vi "Read AI.vi"(8 "error in":errorcluster, 11 "DAQmx in":refnum<class "DAQmx.lvclass">) -> (0 "error out":errorcluster, 2 "AI []":waveform(dbl)[](array[waveform]), 3 "DAQmx out":refnum<class "DAQmx.lvclass">, 4 "AI time (ms)":u32=2)   [LabVIEW 2019, in "DAQmx.lvclass"]
uses:
  DAQmx.lvclass
  <resource>/objmgr/daqmx.rc
  Instrument.DAQ/Instrument.DAQ.lvclass
  Instrument.DAQ/Waveguide Model/Waveguide Model--Cluster.ctl
  <vilib>/Waveform/WDTOps.llb/WDT Append Waveforms DBL.vi
  <vilib>/DAQmx/read.llb/DAQmx Read (Analog 1D Wfm NChan NSamp).vi
panel:
  out "Available Samples":u32[][](graph)
  in  "show graph?":bool
  out "Ratio Chart":u32[][](graph)
  out "Waveform Graph":waveform(dbl)[](graph)
  out "P Check":bool[](array[boolean])
  out "Numeric":i32
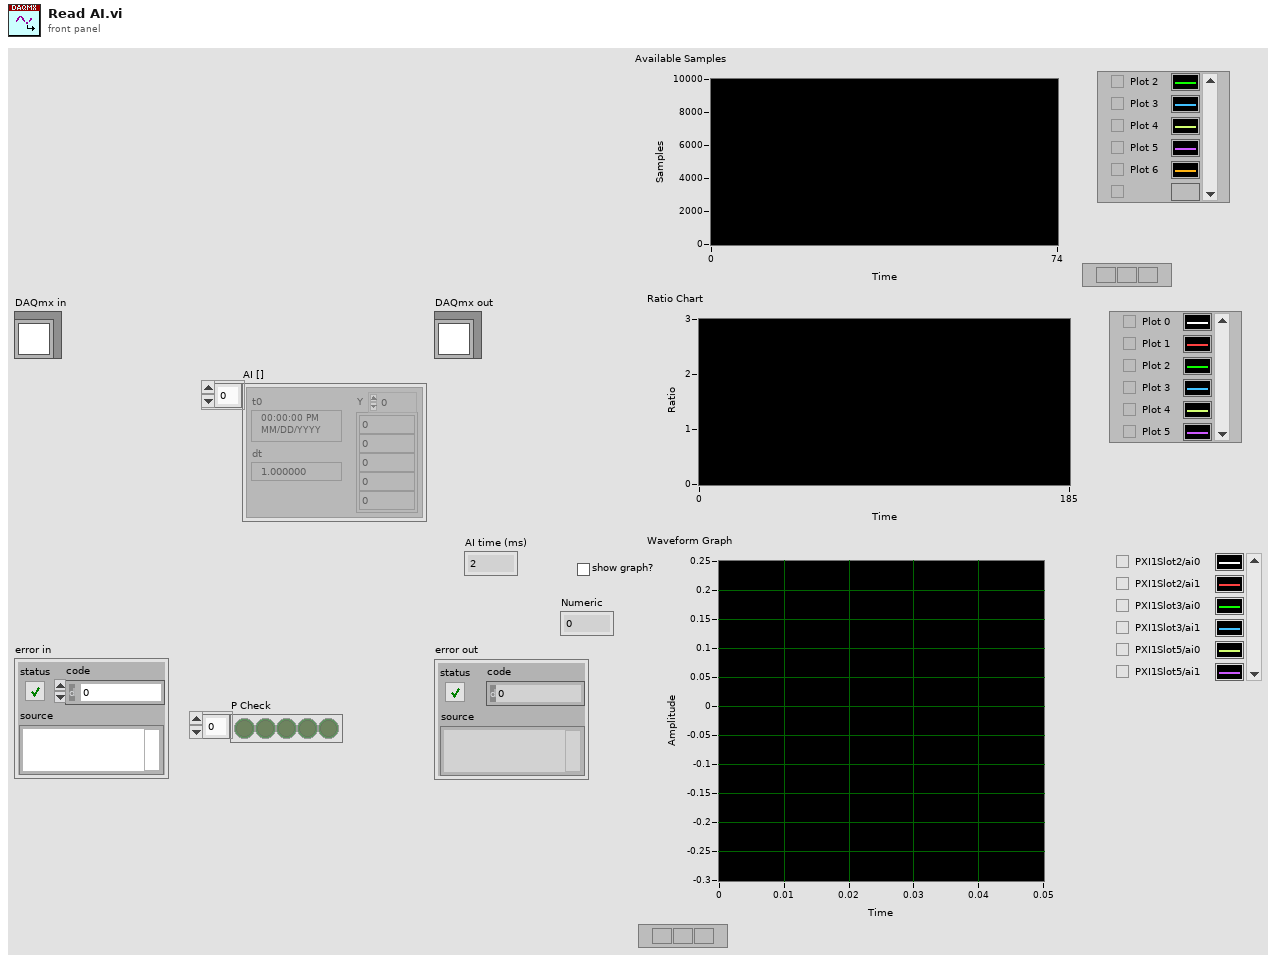
[diagram p1: front panel]
types:
  T1 = typedef "Instrument.Lockin.lvlib/Instrument.DAQ.lvclass/Waveguide Model--Cluster.ctl" = cluster{"Vsource Index":i32, "Vsg Index":i32, "V+":i32, "V-":i32}
  T2 = typedef "DAQmx.lvclass/DAQ.Config.AI--Cluster--Array.ctl" = T3[]
  T3 = typedef "DAQmx.lvclass/DAQ.Config.AI--Cluster.ctl" = cluster{"Channels":tag, "Coupling":T4, "Range":T5, "input terminal configuration":i32, "Type":T6}
  T4 = typedef "DAQmx.lvclass/DAQ.Config.AI.Coupling--enum.ctl" = u16
  T5 = typedef "DAQmx.lvclass/DAQ.Config.AI.Range--enum.ctl" = enum16{"±0.316", "±1.00", "±3.16", "±10.0", "±31.6", "±42.4", ""}
  T6 = typedef "DAQmx.lvclass/DAQ.Config.Device Type--enum.ctl" = enum16{"None", "USB-4431", "PXI-446x"}
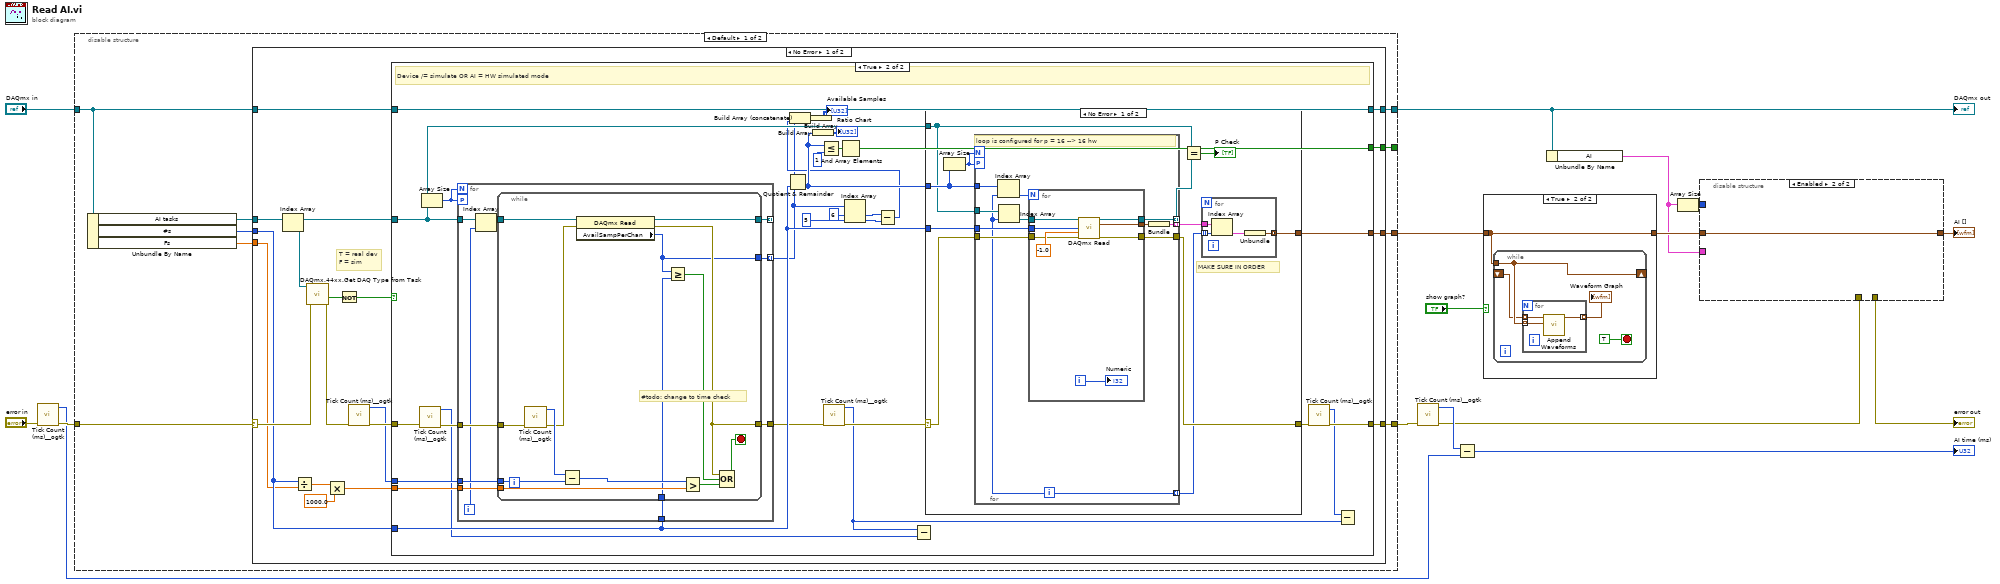
[diagram p0: block diagram]
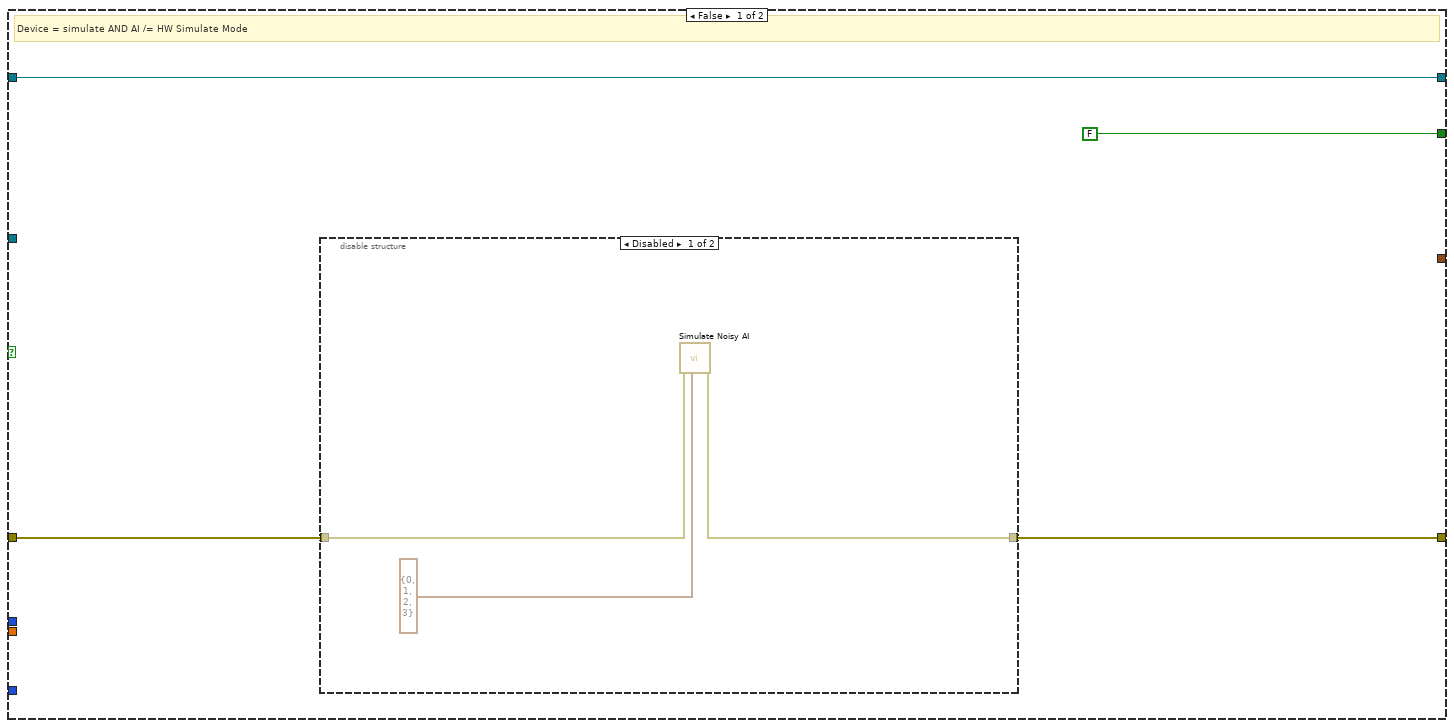
[diagram p2: hidden frame]
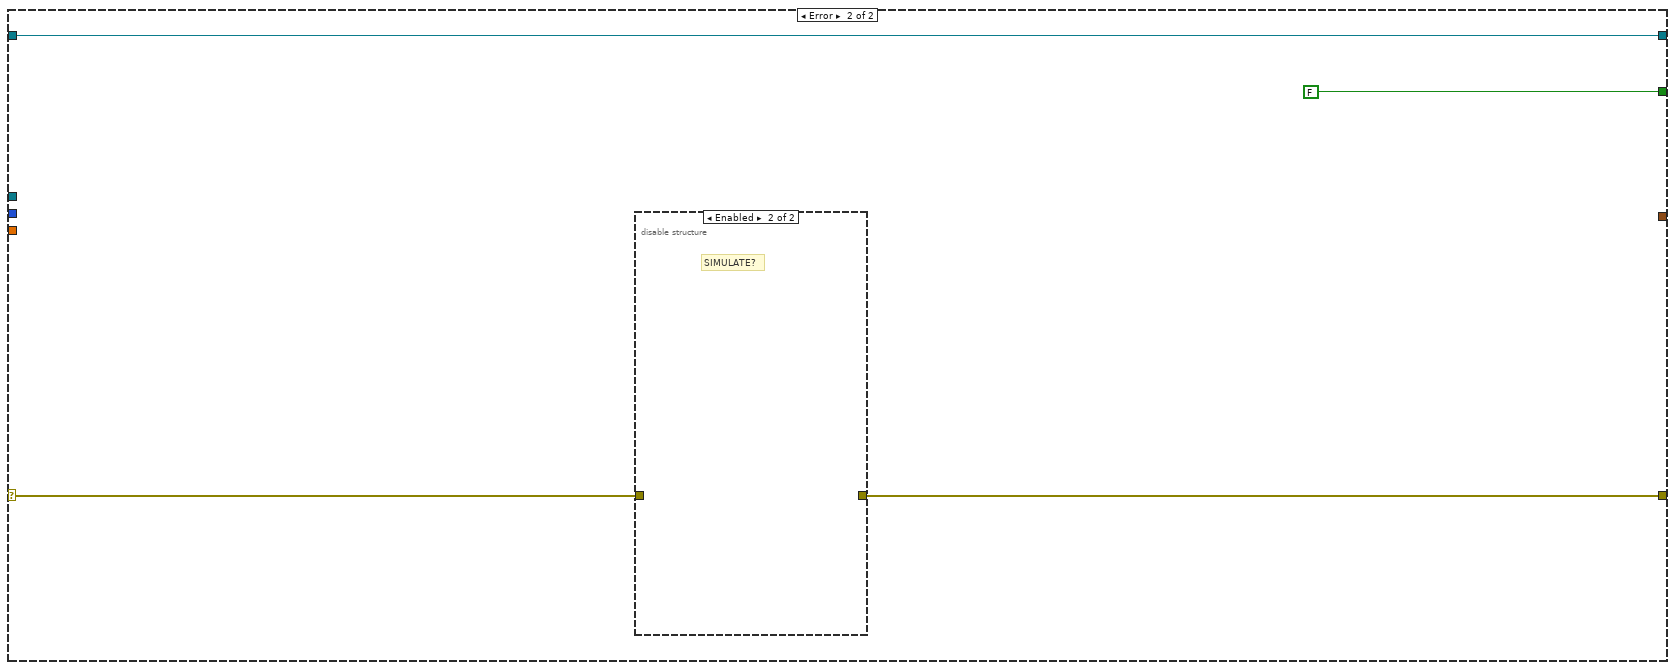
[diagram p5: hidden frame]
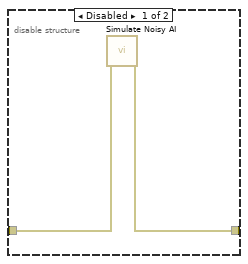
[diagram p6: hidden frame]
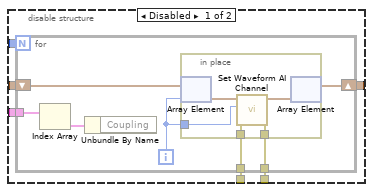
[diagram p8: hidden frame]
diagram:
  n1 = call <userlib>:"Tick Count (ms)__ogtk.vi"("error in (no error)"="error in") -> ("error out"=w15:errorcluster, "millisecond timer value"=w11:u32)  [unwired: 9 in]
  n2 = disable-structure shown="Default" {
    disable-tunnel: [w24 w146] -> w10
    disable-tunnel: "DAQmx in" -> [w23 w145]
    disable-tunnel: w15 -> [w20 w146]
    disable-tunnel: [w22 w145] -> w2
    disable-tunnel: [w19 _] -> _
    disable-tunnel: [w18 _] -> w3
    frame condition #0 (active) {
      n3 = Unbundle By Name(w23) -> ("AI tasks"=w21:refnum<k21>[], "#s"=w25:i32, "Fs"=w17:dbl)
      n4 = case shown="No Error" w20 {
        selector: w20 -> [w41 w141]
        tunnel: w25 -> [w40 _]
        tunnel: [w42 w142] -> w24
        tunnel: w21 -> [w32 _]
        tunnel: w23 -> [w43 w139]
        tunnel: [w30 w139] -> w22
        tunnel: w17 -> [w39 _]
        tunnel: [w29 FALSE] -> w19
        tunnel: [w28 _] -> w18
        frame No Error {
          # "T = real dev\nF = sim"
          n5 = Index Array(array=w32) -> (element=w26:refnum<k21>)  [unwired: 1 in]
          n6 = Divide(x=w40, y=w39) -> (x/y=w38:dbl)
          n7 = call "DAQmx.44xx.Get DAQ Type from Task.vi"("error in (no error)"=w41, "Task in"=w26) -> ("error out"=w35:errorcluster, "DevIsSimulated"=w31:bool)  [unwired: 6 in, 2 out]
          n8 = Multiply(x=w38, y=1000.0) -> (x*y=w34:dbl)
          n9 = Not(x=w31) -> (.not. x?=w27:bool)
          n10 = call <userlib>:"Tick Count (ms)__ogtk.vi"("error in (no error)"=w35) -> ("error out"=w36:errorcluster, "millisecond timer value"=w33:u32)  [unwired: 9 in]
          n11 = case shown="True" w27 {
            tunnel: w40 -> [_ w79]
            tunnel: w36 -> [w47 w77]
            tunnel: [w46 w78] -> w42
            tunnel: w43 -> [w44 w52]
            tunnel: w34 -> [_ w76]
            tunnel: w33 -> [_ w75]
            tunnel: w32 -> [_ w74]
            tunnel: [w44 w52] -> w30
            tunnel: [FALSE w73] -> w29
            tunnel: [_ w51] -> w28
            frame False {
              # "Device = simulate AND AI /= HW Simulate Mode"
              n12 = disable-structure shown="Disabled" {
                disable-tunnel: w47 -> [w49 _]
                disable-tunnel: [w48 _] -> w46
                frame Disabled {
                  n13 = call "Simulate Noisy AI.vi"("Waveguide Cluster"=T1 {"Vsource Index"=0, "Vsg Index"=1, "V+"=2, "V-"=3}, "error in (no error)"=w49) -> ("error out"=w48:errorcluster)  [unwired: 7 in, 2 out]
                }
                frame Enabled {
                  # "SIMULATE"
                }
              }
            }
            frame True {
              # "Device /= simulate OR AI = HW simulated mode"
              n14 = call <userlib>:"Tick Count (ms)__ogtk.vi"("error in (no error)"=w77) -> ("error out"=w72:errorcluster, "millisecond timer value"=w68:u32)  [unwired: 9 in]
              n15 = Array Size(array=w74) -> (size(s)=w65:i32)
              n16 = for {
                N: w65 -> [_]
                tunnel: w79 -> [w89]
                tunnel: w76 -> [w87]
                tunnel: w74 -> [w81]
                tunnel: w75 -> [w84]
                tunnel: [w86] -> w53 mode=indexing
                tunnel: [w83] -> _ mode=indexing
                workers-P: w65 -> [_]
                tunnel: w72 -> [w88]
                tunnel: [w85] -> w71
                i -> [w80]
                n17 = Index Array(array=w81, index=w80) -> (element=w82:refnum<k21>)
                n18 = while {
                  tunnel: [w103] -> w83
                  tunnel: w88 -> [w98]
                  tunnel: [w101] -> w85
                  tunnel: w89 -> [w92]
                  tunnel: w87 -> [w99]
                  tunnel: [w93] -> w86
                  tunnel: w84 -> [w96]
                  tunnel: w82 -> [w91]
                  stop <- w102 stop-if-true
                  # "#todo: change to time check"
                  n19 = call <userlib>:"Tick Count (ms)__ogtk.vi"("error in (no error)"=w98) -> ("error out"=w90:errorcluster, "millisecond timer value"=w97:u32)  [unwired: 9 in]
                  n20 = Subtract(x=w97, y=w96) -> (x-y=w95:u32)
                  n21 = property class="DAQmx Read"(reference=w91, error in=w90) -> (reference out=w103:refnum<k21>, error out=w101:errorcluster, "AvailSampPerChan"=w93:u32)
                  n22 = Greater Or Equal?(x=w93, y=w92) -> (x >= y?=w94:bool)
                  n23 = Greater?(x=w95, y=w99) -> (0:w100:bool)
                  n24 = Compound Arithmetic op=OR(w101, w94, w100) -> (w102:bool)
                }
              }
              n25 = Quotient & Remainder(x=w53, y=w79) -> (floor(x/y)=w61:u32[])  [unwired: 1 out]
              n26 = Build Array(w61) -> (→"Ratio Chart":u32[][])
              n27 = Less Or Equal?(x=w61, y=u32 1) -> (x <= y?=w63:bool[])
              n28 = call <userlib>:"Tick Count (ms)__ogtk.vi"("error in (no error)"=w71) -> ("error out"=w70:errorcluster, "millisecond timer value"=w66:u32)  [unwired: 9 in]
              n29 = And Array Elements(Boolean array=w63) -> (logical AND=w73:bool)
              n30 = Index Array(array=w53, index #1=6 ("index"), index #2=5 ("index")) -> (element #1=w57:u32, element #2=w56:u32)
              n31 = Subtract(x=w57, y=w56) -> (x-y=w55:u32)
              n32 = Build Array (concatenate)(w53, w55) -> (w60:u32[])
              n33 = Build Array(w60) -> (→"Available Samples":u32[][])
              n34 = Subtract(x=w66, y=w68) -> ()  [unwired: 1 out]
              n35 = case shown="No Error" w70 {
                selector: w70 -> [w113 w138]
                tunnel: [w106 _] -> w51
                tunnel: w79 -> [w114 _]
                tunnel: [w111 w138] -> w69
                tunnel: w61 -> [w112 _]
                tunnel: w74 -> [w110 _]
                frame No Error {
                  # "MAKE SURE IN ORDER"
                  n36 = Array Size(array=w112) -> (size(s)=w104:i32)
                  n37 = for {
                    N: w104 -> [_]
                    tunnel: w114 -> [w125]
                    tunnel: [w121] -> w107 mode=indexing
                    tunnel: w112 -> [w117]
                    tunnel: w113 -> [w123]
                    tunnel: [w122] -> w111
                    tunnel: w110 -> [w118]
                    workers-P: w104 -> [_]
                    tunnel: [w116] -> w108 mode=indexing
                    tunnel: [w120] -> w105 mode=indexing
                    i -> [w116]
                    # "loop is configured for p = 16 --> 16 hw"
                    n38 = Index Array(array=w117, index=w116) -> (element=w115:u32)
                    n39 = Index Array(array=w118, index=w116) -> (element=w119:refnum<k21>)
                    n40 = for {
                      N: w115 -> [_]
                      tunnel: w119 -> [w126]
                      tunnel: w123 -> [w127]
                      tunnel: [w133] -> w124
                      tunnel: w125 -> [w128]
                      tunnel: [w132] -> w122
                      tunnel: [w129] -> w120
                      i -> [w131]
                      n41 = call-poly <vilib>:"DAQmx Read.vi"("task/channels in"=w126, "number of samples per channel"=w128, "timeout"=-1.0, "error in"=w127) -> ("task out"=w129:refnum<k21>, "data"=w133:waveform(dbl)[], "error out"=w132:errorcluster)  [unwired: 9 in]
                      "Numeric" <- w131
                    }
                    n42 = Bundle("data"=w124) -> (w121:cluster{"data":waveform(dbl)[]})  [unwired: 1 in]
                  }
                  n43 = Equal?(x=w110, y=w105) -> (x = y?=→"P Check":bool[])
                  n44 = for {
                    tunnel: w108 -> [w137] mode=indexing
                    tunnel: w107 -> [w136]
                    tunnel: [w135] -> w106 mode=concatenating
                    n45 = Index Array(array=w136, index=w137) -> (element=w134:cluster{"data":waveform(dbl)[]})
                    n46 = Unbundle(w134) -> ("data"=w135:waveform(dbl)[])
                  }
                }
                frame Error {
                }
              }
              n47 = call <userlib>:"Tick Count (ms)__ogtk.vi"("error in (no error)"=w69) -> ("error out"=w78:errorcluster, "millisecond timer value"=w67:u32)  [unwired: 9 in]
              n48 = Subtract(x=w67, y=w66) -> ()  [unwired: 1 out]
            }
          }
        }
        frame Error {
          n49 = disable-structure shown="Enabled" {
            disable-tunnel: [w144 _] -> w142
            disable-tunnel: w141 -> [w143 _]
            frame Disabled {
              n50 = call "Simulate Noisy AI.vi"("error in (no error)"=w143) -> ("error out"=w144:errorcluster)  [unwired: 8 in, 2 out]
            }
            frame Enabled {
              # "SIMULATE?"
            }
          }
        }
      }
    }
    frame condition #1 {
    }
  }
  "DAQmx out" <- w2
  n51 = call <userlib>:"Tick Count (ms)__ogtk.vi"("error in (no error)"=w10) -> ("error out"=w1:errorcluster, "millisecond timer value"=w14:u32)  [unwired: 9 in]
  n52 = Subtract(x=w14, y=w11) -> (x-y=→"AI time (ms)":u32)
  n53 = case shown="True" "show graph?" {
    tunnel: w3 -> [w147 w148]
    tunnel: [w147 w148] -> w8
    frame False {
    }
    frame True {
      n54 = while {
        shift-right: [w150] -> _
        shift-left: _ -> [w149]
        tunnel: w148 -> [w150]
        stop <- TRUE stop-if-true
        n55 = for {
          tunnel: [w155] -> w151 mode=indexing
          tunnel: w149 -> [w154] mode=indexing
          tunnel: w150 -> [w153] mode=indexing
          n56 = call-poly <vilib>:"Append Waveforms.vi"("waveform B"=w153, "waveform A"=w154) -> ("waveform out"=w155:waveform(dbl))  [unwired: 8 in, 1 out]
        }
        "Waveform Graph" <- w151
      }
    }
  }
  n57 = Unbundle By Name(w2) -> ("AI"=w5:T2)
  n58 = Array Size(array=w5) -> (size(s)=w4:i32)
  n59 = disable-structure shown="Enabled" {
    disable-tunnel: w8 -> [w161 w174]
    disable-tunnel: w1 -> [w160 _]
    disable-tunnel: [w159 _] -> w7
    disable-tunnel: [w158 w174] -> w6
    disable-tunnel: w5 -> [w157 _]
    disable-tunnel: w4 -> [w156 _]
    frame Disabled {
      n60 = for {
        N: w156 -> [_]
        tunnel: w157 -> [w163]
        tunnel: w160 -> [w167]
        tunnel: [w166] -> w159
        shift-right: [w165] -> w158
        shift-left: w161 -> [w168]
        i -> [w162]
        n61 = Index Array(array=w163) -> (element=w164:T3)  [unwired: 1 in]
        n62 = Unbundle By Name(w164) -> ()  [unwired: 1 out]
        n63 = in-place {
          in-place-border: w167 -> [w171]
          in-place-border: [w170] -> w166
          in-place-border: w162 -> [w169]
          n64 = in-place-array #1(w168, w162) -> (w173:waveform(dbl))
          n65 = call "Set Waveform AI Channel.vi"("error in (no error)"=w171, "AI Channel"=w169, "Waveform in"=w173) -> ("error out"=w170:errorcluster, "Waveform out"=w172:waveform(dbl))  [unwired: 7 in]
          n66 = in-place-array #1(w172) -> (w165:waveform(dbl)[])  [unwired: 1 out]
        }
      }
    }
    frame Enabled {
    }
  }
  "error out" <- w7
  "AI []" <- w6
